vi "Initialize Window Positions.vi"(8 "error in (no error)":errorcluster, 11 "MainController in":refnum<class "MainController.lvclass">) -> (0 "error out":errorcluster, 3 "MainController out":refnum<class "MainController.lvclass">)   [LabVIEW 2012, in "Win8uiFramework.lvlib" / "MainController.lvclass"]
uses:
  MainController.lvclass
  <vilib>/Utility/miscctls.llb/LVPointTypeDef.ctl
  Visibility Direction.ctl
  MainController.lvclass/MainController.ctl
  Read UI VI Ref.vi
  Read Main Pane.vi
  Read Active SubPanel.vi
  Win8uiFramework.lvlib
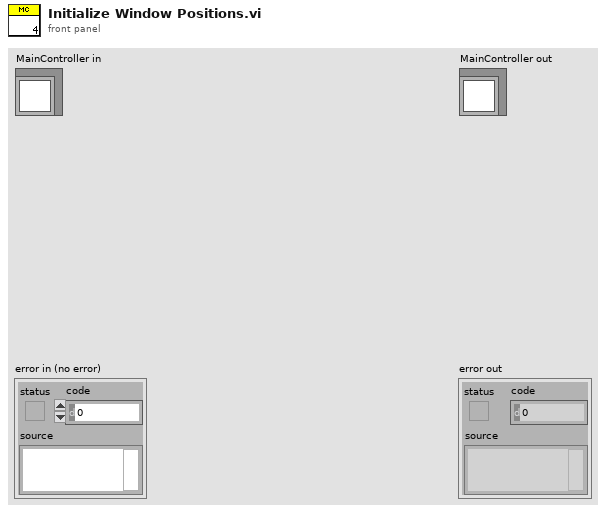
[diagram p1: front panel]
types:
  T1 = typedef "Win8uiFramework.lvlib/Visibility Direction.ctl" = enum16{"Show", "Hide"}
  T2 = typedef "LVPointTypeDef.ctl" = cluster{"Horizontal":i16, "Vertical":i16}
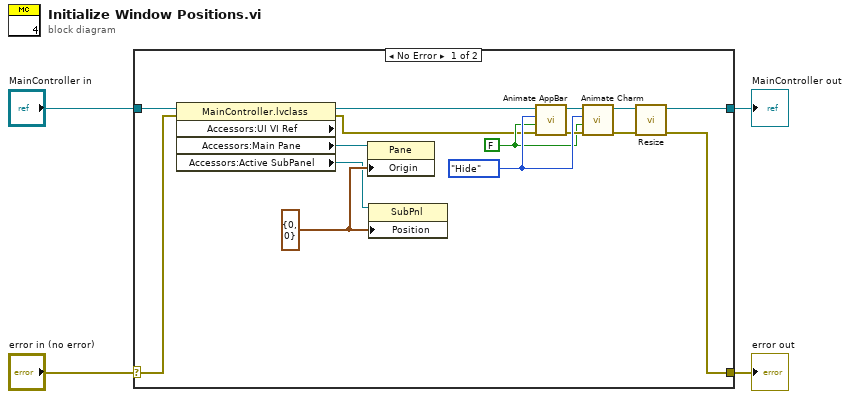
[diagram p0: block diagram]
diagram:
  n1 = case shown="No Error" "error in (no error)" {
    selector: "error in (no error)" -> [w14 w21]
    tunnel: [w9 w21] -> w3
    tunnel: [w7 w20] -> w1
    tunnel: "MainController in" -> [w19 w20]
    frame No Error {
      w13 = FALSE ("Smooth?")
      w16 = Visibility_Direction."Hide" ("Direction")
      w6 = T2 {"Horizontal"=0, "Vertical"=0} ("Origin")
      n2 = property class="MainController.lvclass" props=["Accessors:UI VI Ref", "Accessors:Main Pane", "Accessors:Active SubPanel"](reference=w19, error in=w14) -> (reference out=w12:refnum<class "MainController.lvclass">, error out=w11:errorcluster, "Accessors:Main Pane"=w18:refnum<vi>, "Accessors:Active SubPanel"=w5:refnum<vi>)  [unwired: 1 out]
      n3 = property class="Pane"(reference=w18, "Origin"=w6) -> ()  [unwired: 1 in, 2 out]
      n4 = property class="SubPnl"(reference=w5, "Position"=w6) -> ()  [unwired: 1 in, 2 out]
      n5 = call-dynamic "Animate AppBar.vi"("error in (no error)"=w11, "Smooth?"=w13, "Direction"=w16, "MainController in"=w12) -> ("error out"=w15:errorcluster, "MainController out"=w17:refnum<class "MainController.lvclass">)  [unwired: 6 in]
      n6 = call-dynamic "Animate Charm.vi"("error in (no error)"=w15, "Smooth?"=w13, "Direction"=w16, "MainController in"=w17) -> ("error out"=w10:errorcluster, "MainController out"=w8:refnum<class "MainController.lvclass">)  [unwired: 6 in]
      n7 = call "Resize.vi"("error in (no error)"=w10, "MainController in"=w8) -> ("error out"=w9:errorcluster, "MainController out"=w7:refnum<class "MainController.lvclass">)  [unwired: 8 in]
    }
    frame Error {
    }
  }
  "error out" <- w3
  "MainController out" <- w1
